vi "DiscArchiver.write file.vi"(0 "i ref in":refnum<vi>, 2 "eventData":string, 5 "error in (no error)":errorcluster) -> (14 "i ref out":refnum<vi>, 19 "error out":errorcluster)   [LabVIEW 2014, in "DiscArchiver.lvlib"]
doc: "Writes one event (one datum of eventData) to a file. The event data is a byte array."
uses:
  DiscArchiver.lvlib
  CSCore/CSSystem/CoreDefs/CoreDefs.error_type.ctl
  CSCore/CSSystem/CoreLib/CoreLib.string 2 byte array.vi
  CSCore/CSSystem/CoreLib/CoreLib.lvlib
  CSlibraries/UtilityLib/UtilityLib.lvlib
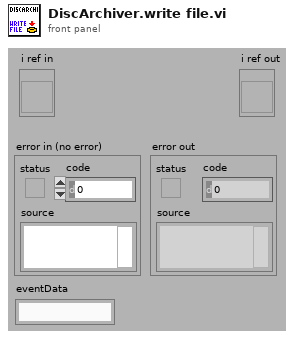
[diagram p1: front panel]
types:
  T1 = typedef "CoreDefs.error_type.ctl" = enum16{"no error", "can't load process", "can't unload process", "process does not exist", "can't install process", "can't remove process", "unknown function", "time out", "can't execute function", "duplicate queue name", "super not found", "caller queue invalid", "can't ping process", "unknown error", "VISA Error", "VISA timeout", "GPIB timeout", "GPIB error", "communication error", "data type mismatch", "can't read data from OPC server", "can't write data to OPC server", "OET error", "function not implemented", "process already exists", "invalid Shared Variable name", "error writing Shared Variable", "error reading Shared Variable", "invalid client name", "corrupt database", "unknown class", "call not authorized", "parameter out of range", "OET timeout: can't get data to modify", "invalid queue name", "requested operation incompatible with current state", "event undefined", "event disabled", "state undefined", "caller is not a friend", "EventBuilder: bad eventID", "EventBuilder: no DAQ devices", "a thread must not stop itself", "UNUSED ELEMENT4", "DiscArchiver: eventData incomplete", "DiscArchiver: eventData does not belong to run", "DiscArchiver: can't open file", "DiscArchiver: can't write to file", "DiscArchiver: available disc space low", "can't acquire semaphore", "error reading data from database", "notifier object is not existing", "can't register process", "can't unregister process", "illegal event type", "object disabled", "object already exists", "can't change state", "Instrument not found", "no connection to remote node", "invalid reference", "N/A", "UNUSED ELEMENT 1", "element not found", "illegal TCP/IP connection detected", "object does not exist", "invalid access ID", "unknown CS system", "invalid privilige", "unsupported data type", "unsupported server type", "IO server already exists", "Shared Variable already exists"}
  T2 = typedef "DiscArchiver.lvlib/DiscArchiver.i attribute.ctl" = cluster{"file prefix":string, "actual file":string, "nOfEvents":i32, "file":refnum<file>, "eventBuilder":string, "disc size alarm":bool, "dataDescription":string, "dataDescriptionURL":string, "eventDataURL":string, "headerID":dbl, "completeData":bool, "nOfEventsID":i32, "dataFileID":i32}
  T3 = typedef "CoreDefs.rawDataType.ctl" = i8[]
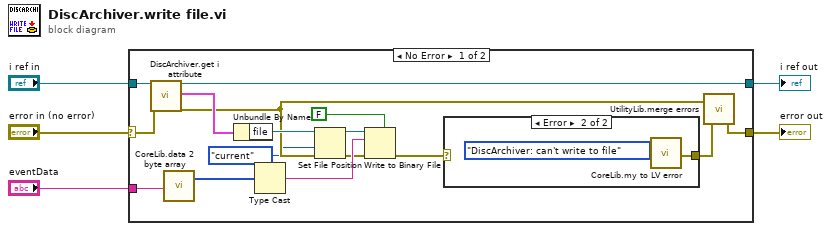
[diagram p0: block diagram]
diagram:
  n1 = case shown="No Error" "error in (no error)" {
    selector: "error in (no error)" -> [w11 w25]
    tunnel: "i ref in" -> [w21 w26]
    tunnel: "eventData" -> [w19 _]
    tunnel: [w17 w26] -> w3
    tunnel: [w15 w25] -> w2
    frame No Error {
      n2 = call "DiscArchiver.get i attribute.vi"("i ref in"=w21, "error in (no error)"=w11) -> ("i ref out"=w17:refnum<vi>, "i attribute"=w20:T2, "error out"=w16:errorcluster)  [unwired: 15 in]
      n3 = call-poly "CoreLib.data 2 byte array.vi"("string"=w19) -> ("byteArray out"=w9:T3)  [unwired: 18 in]
      n4 = Unbundle By Name(w20) -> ("file"=w18:refnum<file>)
      n5 = Type Cast(x=w9) -> (*(type *) &x=w10:string)  [unwired: 1 in]
      n6 = Set File Position(refnum=w18, from (0:start)=enum16{"start", "end", "current"}."current" ("pos mode (0:2)"), error in=w16) -> (refnum out=w8:refnum<file>, error out=w7:errorcluster)  [unwired: 1 in]
      n7 = Write to Binary File(file (use dialog)=w8, data=w10, error in=w7, 5:FALSE ("prepend array or string size? (T)")) -> (error out=w13:errorcluster)  [unwired: 2 in, 2 out]
      n8 = case shown="Error" w13 {
        selector: w13 -> [w22 _]
        tunnel: [w22 w24] -> w12
        frame No Error {
        }
        frame Error {
          n9 = call "CoreLib.my to LV error.vi"("ErrorTypes"=CoreDefs.error_type."DiscArchiver: can't write to file") -> ("myErrorCluster"=w24:errorcluster)  [unwired: 17 in, 1 out]
        }
      }
      n10 = call "UtilityLib.merge errors.vi"("error2 (no error)"=w12, "error1 (no error)"=w16) -> ("error out"=w15:errorcluster)
    }
    frame Error {
    }
  }
  "error out" <- w2
  "i ref out" <- w3
